vi "LakeShore218_init.vi"(11 "VISA in":refnum<visa-resource-name>) -> (0 "error out":errorcluster, 3 "VISA out":refnum<visa-resource-name>, 4 "status":bool)   [LabVIEW 2019]
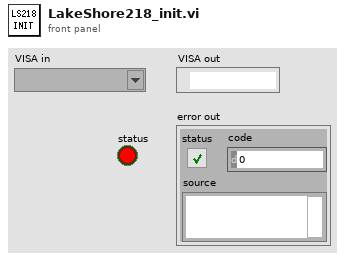
[diagram p1: front panel]
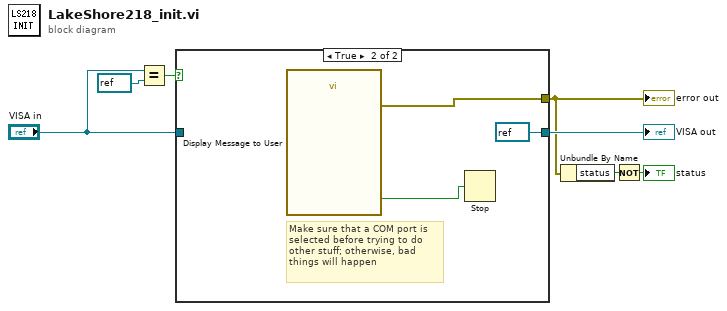
[diagram p0: block diagram]
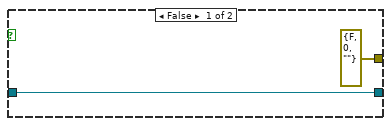
[diagram p2: hidden frame]
diagram:
  n1 = Equal?(x="VISA in", y=refnum<visa-resource-name> refnum) -> (x = y?=w5:bool)
  n2 = case shown="True" w5 {
    tunnel: "VISA in" -> [w9 _]
    tunnel: [w9 refnum<visa-resource-name> refnum ("COM Port")] -> w7
    tunnel: [errorcluster {"status"=FALSE, "code"=0, "source"=""} ("error out") w10] -> w3
    frame False {
    }
    frame True {
      # "Make sure that a COM port is\nselected before trying to do\nother stuff; otherwise, bad\nthings will happen"
      n3 = call "Display Message to User"() -> ("error out"=w10:errorcluster, "OK"=w11:bool)  [unwired: 10 in]
      n4 = Stop(stop? (T)=w11) -> ()
    }
  }
  "VISA out" <- w7
  "error out" <- w3
  n5 = Unbundle By Name(w3) -> ("status"=w2:bool)
  n6 = Not(x=w2) -> (.not. x?=→"status":bool)
